vi "setF_NW.vi"(8 "U_Tor":fxp<+/-,25,5>, 9 "U_ThY":fxp<+/-,25,5>, 10 "U_ThX":fxp<+/-,25,5>, 11 "U_Z":fxp<+/-,25,5>) -> (3 "F_NW out":fxp<+/-,25,5> format="%#.10g")   [LabVIEW 2020, in "CtrlEff.lvlib"]
doc: "Sets the absolute value of the force actuation value for the NW electrode."
uses:
  CtrlEff.lvlib
  <vilib>/Platform/TimedLoop/XDataNode/timing_clust.ctl
  <vilib>/Platform/TimedLoop/XDataNode/nitl_modes.ctl
  <vilib>/Platform/TimedLoop/XDataNode/wakeup.ctl
  <vilib>/rvi/Emulation/niFpgaSctlEmulationGetInTimedLoop.vi
  <vilib>/rvi/Emulation/niFpgaEmulationReportErrorSimple.vi
  <vilib>/rvi/Emulation/niFpgaGetClockAttributes.vi
  <vilib>/rvi/Emulation/niFpgaCriticalErrorInLSC.vi
  <vilib>/Platform/TimedLoop/XDataNode/XDataNode.xnode
  <vilib>/rvi/FXPMathLib/FxpAdd/XNode/nifxpmath_Add.xnode
  <vilib>/rvi/FXPMathLib/FxpMul/XNode/nifxpmath_Multiplier.xnode
  <vilib>/Platform/TimedLoop/XDataNode/XDNodeRunTimeDep.lvlib
  <vilib>/rvi/FXPMathLib/sim/FxpSim.dll
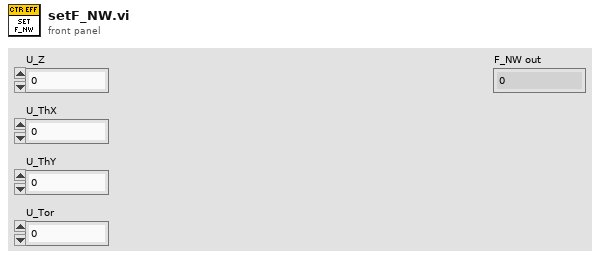
[diagram p1: front panel]
types:
  T1 = typedef "XDNodeRunTimeDep.lvlib/timing_clust.ctl" = cluster{"Expected End [f-1]":u64, "Actual End [f-1]":u64, "Finished Late? [f-1]":bool, "Expected End [i-1]":u64, "Actual End [i-1]":u64, "Finished Late? [i-1]":bool, "Expected Start [i]":u64, "Actual Start [i]":u64, "Expected Start [f]":u64, "Actual Start [f]":u64, "Source Name":string, "Structure Name":string, "Period":i64, "Deadline":i64, "Offset":i64, "Start":i64, "Priority":i32, "Timeout":i32, "Mode":T2, "Wakeup Reason":T3, "Error":errorcluster, "Source Type":string, "Secondary Source Type":string, "Global End Time":u64, "Global Start Time":u64, "Frame Duration":u64, "Iteration Duration":u64, "Assigned CPU":i32, "I/O Scan Engine Mode":u32}
  T2 = typedef "XDNodeRunTimeDep.lvlib/nitl_modes.ctl" = enum32{"No Change", "Process missed periods, maintain original phase", "Discard missed periods, maintain original phase", "Process missed periods, ignore original phase", "Discard missed periods, ignore original phase"}
  T3 = typedef "XDNodeRunTimeDep.lvlib/wakeup.ctl" = enum32{"Normal", "Aborted", "Asynchronous wakeup", "Timing source error", "Timed loop error", "Timeout"}
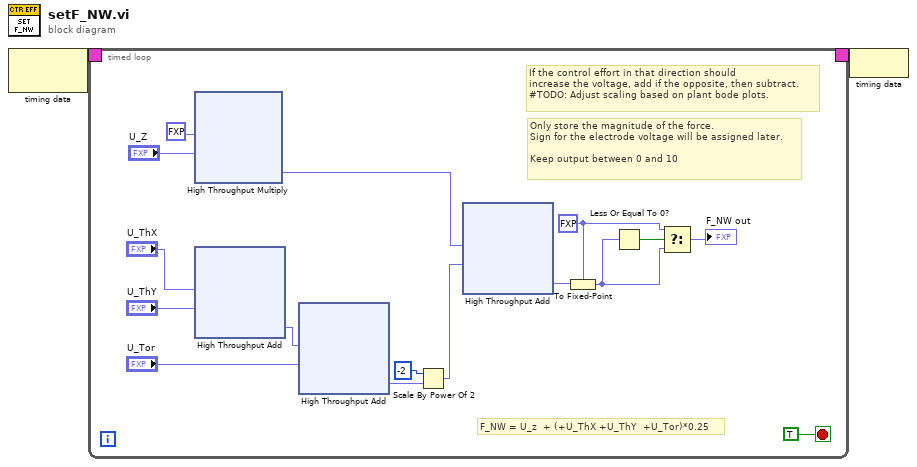
[diagram p0: block diagram]
diagram:
  n1 = node-c288() -> (w2:T1)  [unwired: 1 in]
  n2 = timed-loop {
    timing: w2 -> [_]
    timing-out: [_] -> w1
    stop <- TRUE stop-if-true
    w10 = fxp<+/-,25,5> 0.0 ("t")
    # "F_NW = U_z  + (+U_ThX +U_ThY  +U_Tor)*0.25"
    # "If the control effort in that direction should\nincrease the voltage, add if the opposite, then subtract.\n#TODO: Adjust scaling based on plant bode plots."
    # "Only store the magnitude of the force. \nSign for the electrode voltage will be assigned later.\n\nKeep output between 0 and 10"
    n3 = xnode ("High Throughput Multiply")("x"=fxp<+,1,1> 1.0, "y"="U_Z") -> ("x*y"=w4:fxp<+/-,25,5>)
    n4 = xnode ("High Throughput Add")("x"="U_ThX", "y"="U_ThY") -> ("x+y"=w8:fxp<+/-,26,6>)
    n5 = xnode ("High Throughput Add")("x"=w8, "y"="U_Tor") -> ("x+y"=w9:fxp<+/-,27,7>)
    n6 = Scale By Power Of 2(n=i16 -2, x=w9) -> (x*2^n=w5:fxp<+/-,27,7>)
    n7 = xnode ("High Throughput Add")("x"=w4, "y"=w5) -> ("x+y"=w3:fxp<+/-,28,8>)
    n8 = To Fixed-Point(fixed-point type=w10, number=w3) -> (fixed-point=w11:fxp<+/-,25,5>)
    n9 = Less Or Equal To 0?(x=w11) -> (x <= 0?=w13:bool)
    n10 = Select(t=w10, s=w13, f=w11) -> (s? t:f=→"F_NW out":fxp<+/-,25,5>)
  }
  n11 = node-c288(w1) -> ()
